vi "Initialize Error Log.vi"(0 "Session Handle in":T1, 5 "Error Path":path, 7 "Max File Size":i64, 11 "error in (no error)":errorcluster) -> (4 "Session Handle out":T1, 15 "error out":errorcluster)   [LabVIEW 2015, in "Circular Error Log.lvclass"]
uses:
  Circular Error Log.lvclass
  Typedefs/Session Handle.ctl
  Circular Error Log.lvclass/Circular Error Log.ctl
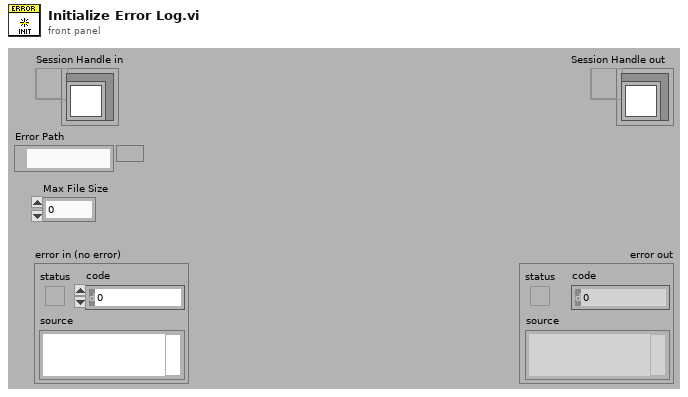
[diagram p1: front panel]
types:
  T1 = typedef "Circular Error Log.lvclass/Session Handle.ctl" = refnum<data-value>
  T2 = enum16{"open", "replace", "create", "open or create", "replace or create", "replace or create with confirmation"}
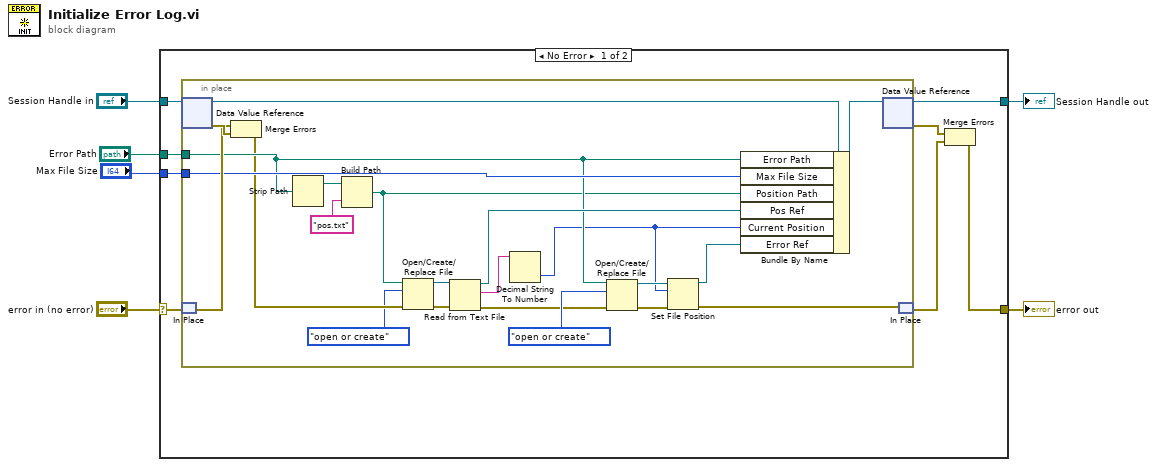
[diagram p0: block diagram]
diagram:
  n1 = case shown="No Error" "error in (no error)" {
    selector: "error in (no error)" -> [w9 w37]
    tunnel: "Session Handle in" -> [w14 w38]
    tunnel: [w13 w38] -> w5
    tunnel: [w10 w37] -> w4
    tunnel: "Error Path" -> [w8 _]
    tunnel: "Max File Size" -> [w7 _]
    frame No Error {
      n2 = in-place {
        in-place-border: w8 -> [w25]
        in-place-border: w7 -> [w28]
        n3 = in-place-dvr #1(w14) -> (w34:refnum<class "Circular Error Log.lvclass">, w36:errorcluster)
        n4 = in-place-match #2(w9) -> (w35:errorcluster)
        n5 = Merge Errors(w35, w36) -> (w19:errorcluster)
        n6 = Strip Path(path=w25) -> (stripped path=w32:path)  [unwired: 1 out]
        n7 = Build Path(base path=w32, name or relative path="pos.txt") -> (appended path=w18:path)
        n8 = Open/Create/Replace File(file path (use dialog)=w18, error in=w19, operation (0:open)=T2."open or create") -> (refnum out=w16:refnum<file>, error out=w15:errorcluster)  [unwired: 3 in, 1 out]
        n9 = Read from Text File(file (use dialog)=w16, error in=w15) -> (refnum out=w29:refnum<file>, text=w30:string, error out=w26:errorcluster)  [unwired: 2 in, 1 out]
        n10 = Decimal String To Number(string=w30) -> (number=w22:i32)  [unwired: 2 in, 1 out]
        n11 = Open/Create/Replace File(file path (use dialog)=w25, error in=w26, operation (0:open)=T2."open or create") -> (refnum out=w23:refnum<file>, error out=w24:errorcluster)  [unwired: 3 in, 1 out]
        n12 = Set File Position(offset (in bytes) (0)=w22, refnum=w23, error in=w24) -> (refnum out=w21:refnum<file>, error out=w20:errorcluster)  [unwired: 1 in]
        n13 = Bundle By Name(cluster=w34, "Error Path"=w25, "Max File Size"=w28, "Position Path"=w18, "Pos Ref"=w29, "Current Position"=w22, "Error Ref"=w21) -> (w33:refnum<class "Circular Error Log.lvclass">)
        n14 = in-place-dvr #1(w33) -> (w13:T1, w11:errorcluster)
        n15 = in-place-match #2(w20) -> (w12:errorcluster)
      }
      n16 = Merge Errors(w11, w12) -> (w10:errorcluster)
    }
    frame Error {
    }
  }
  "Session Handle out" <- w5
  "error out" <- w4
